vi "populate_config_combos.vi"(8 "error in (no error)":errorcluster, 9 "plug-in path refs":refnum<vi>[](array[refnum]), 10 "combo control refs":refnum<vi>[](array[refnum]), 11 "configurations":T1[](array[typedef])) -> (0 "error out":errorcluster)   [LabVIEW 2010]
uses:
  clusters/plugin_specification.ctl
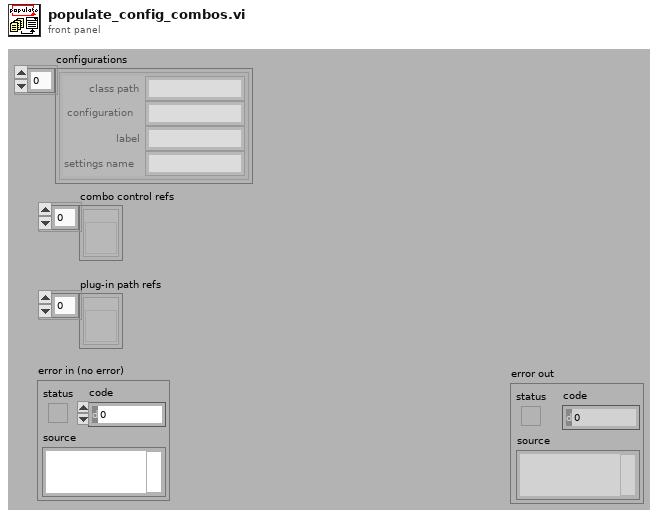
[diagram p1: front panel]
types:
  T1 = typedef "plugin_specification.ctl" = cluster{"class path":string, "configuration":string, "label":string, "settings name":string}
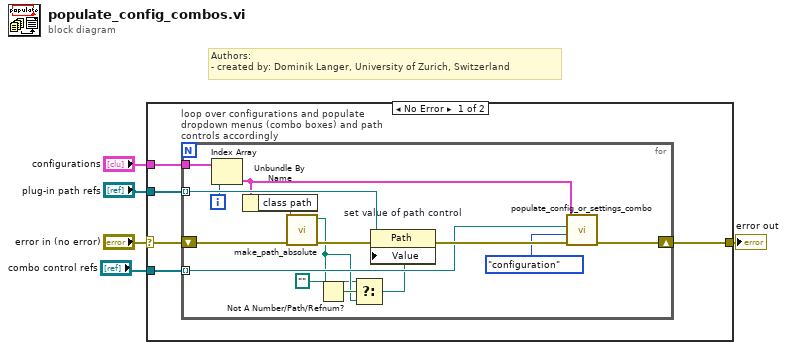
[diagram p0: block diagram]
diagram:
  # "Authors: \n- created by: Dominik Langer, University of Zurich, Switzerland"
  n1 = case shown="No Error" "error in (no error)" {
    selector: "error in (no error)" -> [w10 w26]
    tunnel: [w9 w26] -> w4
    tunnel: "configurations" -> [w8 _]
    tunnel: "combo control refs" -> [w7 _]
    tunnel: "plug-in path refs" -> [w6 _]
    frame No Error {
      n2 = for "loop over configurations and populate dropdown menus (combo boxes) and path controls accordingly" {
        tunnel: w8 -> [w24]
        tunnel: w7 -> [w21] mode=indexing
        tunnel: w6 -> [w25] mode=indexing
        shift-right: [w20] -> w9
        shift-left: w10 -> [w18]
        i -> [w23]
        n3 = Index Array(array=w24, index=w23) -> (element=w11:T1)
        n4 = Unbundle By Name(w11) -> ("class path"=w16:string)
        n5 = call "make_path_absolute.vi"("error in (no error)"=w18, "relative path"=w16) -> ("error out"=w17:errorcluster, "absolute path"=w14:path)  [unwired: 8 in]
        n6 = Not A Number/Path/Refnum?(number/path/refnum=w14) -> (NaN/Path/Refnum?=w15:bool)
        n7 = Select(t=path "", s=w15, f=w14) -> (s? t:f=w13:path)
        n8 = property on="set value of path control" class="Path"(reference=w25, error in=w17, "Value"=w13) -> (error out=w22:errorcluster)  [unwired: 1 out]
        n9 = call "populate_config_or_settings_combo.vi"("error in (no error)"=w22, "type"=enum16{"configuration", "settings"}."configuration", "combo-box reference"=w21, "plug-in specification"=w11) -> ("error out"=w20:errorcluster)  [unwired: 7 in]
      }
    }
    frame Error {
    }
  }
  "error out" <- w4
